vi "Continuous Swept-Sine MeasurementsV2.vi"() -> ()   [LabVIEW 2018]
doc: "Overview:\nThis VI demonstrates simultaneous frequency response, level, and distortion measurements using a discrete swept-sine technique. This example implements analog input and analog output with 'Finite Samples' sample mode which minimizes sensitivity to bandwidth issues that can cause run-time errors when performing continuous measurements. This VI also demonstrates how finite acquisitions can be read in a single large block or in a series of smaller reads.\n\nRequirements:\nLabVIEW Full Development System\nSound and Vibration Toolkit\n\nInstructions:\n1. Connect the DUT to the DSA device.\n2. Select the AO excitation channel, AI stimulus channel, and AI response channel.\n3. Run the VI.\n\nDetails:\nThis VI performs a swept sine measurement to obtain the root-mean-square (RMS) levels of the acquired stimulus and response, the frequency response of the device under test (DUT), and the harmonic distortion on the response channel. You specify the source and measurement parameters, and the swept sine VIs handle all the DAQ-specific controls required to perform the measurement. You have direct control over the source, input, averaging, and display parameters. You also specify the engineering units to use for the swept sine measurements.\n\nYou can view the time records of the acquired stimulus and response signals. From these graphs, you can see that the transition to the next test frequency always occurs at a zero crossing to minimize non-linear disturbances to the DUT. The RMS levels, frequency response, and harmonic distortion are shown on different tabs."
uses:
  <vilib>/sound2/lvsound2.llb/Sampling Mode.ctl
  <vilib>/sound2/lvsound2.llb/Sound Data Format.ctl
  <vilib>/Utility/error.llb/DialogType.ctl
  <vilib>/addons/_NISVFA/_Shared subVIs/Controls/svc_Window.ctl
  <vilib>/addons/_NISVFA/_Generation/Signal Generation/SV Signal/SV Signal.lvclass/SV Signal.ctl
  <vilib>/addons/_NISVFA/_Shared subVIs/Common/svc_Get Waveform Subset (Index).vi
  <vilib>/addons/_NISVFA/_Generation/Signal Generation/SV Signal/Write Leading Synchronization Pulse Enable.vi
  <vilib>/addons/_NISVFA/_Generation/Signal Generation/SV Signal/Write Ramp-Up.vi
  <vilib>/addons/_NISVFA/_Generation/Signal Generation/SV Signal/Write Ramp-Down.vi
  <vilib>/addons/_NISVFA/_Shared subVIs/Common/svc_Get Array Subset (Index).vi
  <vilib>/addons/_NISVFA/_Shared subVIs/Common/svc_Coerce Index and Length.vi
  <vilib>/addons/_NISVFA/_Shared subVIs/Common/svc_Conditional Merge Error.vi
  <vilib>/addons/_NISVFA/_Generation/Signal Generation/SV Continuous Sweep/SV Continuous Sweep.lvclass
  C:/Program Files (x86)/National Instruments/LabVIEW 2018/vi.lib/addons/_NISVFA/_Generation/Signal Generation/SV Signal/SV Signal.lvclass
  <vilib>/addons/_NISVFA/_Generation/Signal Generation/SV Continuous Sweep/Configure Continuous Sweep.vi
  <vilib>/addons/_NISVFA/_Generation/Signal Generation/SV Signal/Write Ramp Parameters.vi
  <vilib>/addons/_NISVFA/_Generation/Signal Generation/SV Signal/Write DC Offset.vi
  <vilib>/addons/_NISVFA/_Generation/Signal Generation/SV Signal/Write Transition Profile.vi
  <vilib>/addons/_NISVFA/_Generation/Signal Generation/SV Signal/Write Pre-Measurement Settling Duration.vi
  <vilib>/addons/_NISVFA/_Generation/Signal Generation/SV Signal/Write Post-Measurement Settling Duration.vi
  <vilib>/sound2/lvsound2.llb/Sound Output Set Volume (Single).vi
  <vilib>/sound2/lvsound2.llb/Sound Output Write (DBL Single).vi
  <vilib>/sound2/lvsound2.llb/Sound Input Read (DBL).vi
  <vilib>/Waveform/WDTOps.llb/WDT Copy Waveform dt DBL.vi
  <vilib>/measure/maresamp.llb/Align N Waveforms (single shot).vi
  <vilib>/addons/_NISVFA/_Baseband FFT/SVFA FFT Spectrum (Complex) (1 Ch).vi
  <vilib>/addons/Sound and Vibration/svt_Single Tone Measurements/SVT Gain and Phase (Frequency).vi
  <vilib>/addons/Sound and Vibration/svt_Distortion/SVT THD and Harmonic Components (Frequency) (1 Ch).vi
  <vilib>/addons/_NISVFA/_Generation/Signal Generation/SV Signal/SV Signal.lvclass
  Program Files (x86)/National Instruments/LabVIEW 2018/examples/Sound and Vibration/SoundVib_Audio Examples.lvlib
  <vilib>/addons/Sound and Vibration/svt_Continuous Swept Sine/SoundVib_ContSweptSine.lvlib
  <vilib>/addons/Sound and Vibration/svt_Distortion/SoundVib_Distortion.lvlib
  <vilib>/addons/Sound and Vibration/svt_Single Tone Measurements/SoundVib_SingleTone.lvlib
  <vilib>/measure/NI_MAPro.lvlib
panel:
  in  "device In":u32
  in  "device Out":u32=1
  out "Magnitude":cluster{"frequency":dbl[], "magnitude":dbl[]}(graph)
  out "Phase":cluster{"frequency":dbl[], "magnitude":dbl[]}(graph)
  out "THD":cluster{"frequency":dbl[], "THD":dbl[]}(graph)
  out "Waveform Graph":waveform(dbl)[](graph)
  out "error aP":errorcluster
  in  "Samples/Sec":dbl=44100.0
  out "test time":u32 format="%.0f ms"
  out "error Mic":errorcluster
  out "error Spkr":errorcluster
  in  "DC offset":dbl format="%.2f V"
  in  "amplitude":dbl=1.0 format="%.2p V"
  in  "frequency range":cluster{"start":dbl, "stop":dbl}={"start"=20000.0, "stop"=40.0} {"stop" min=0.0 format="%.2f Hz"; "start" min=0.0 format="%.2f Hz"}
  in  "duration":dbl=3.0 min=0.0 format="%.2f s"
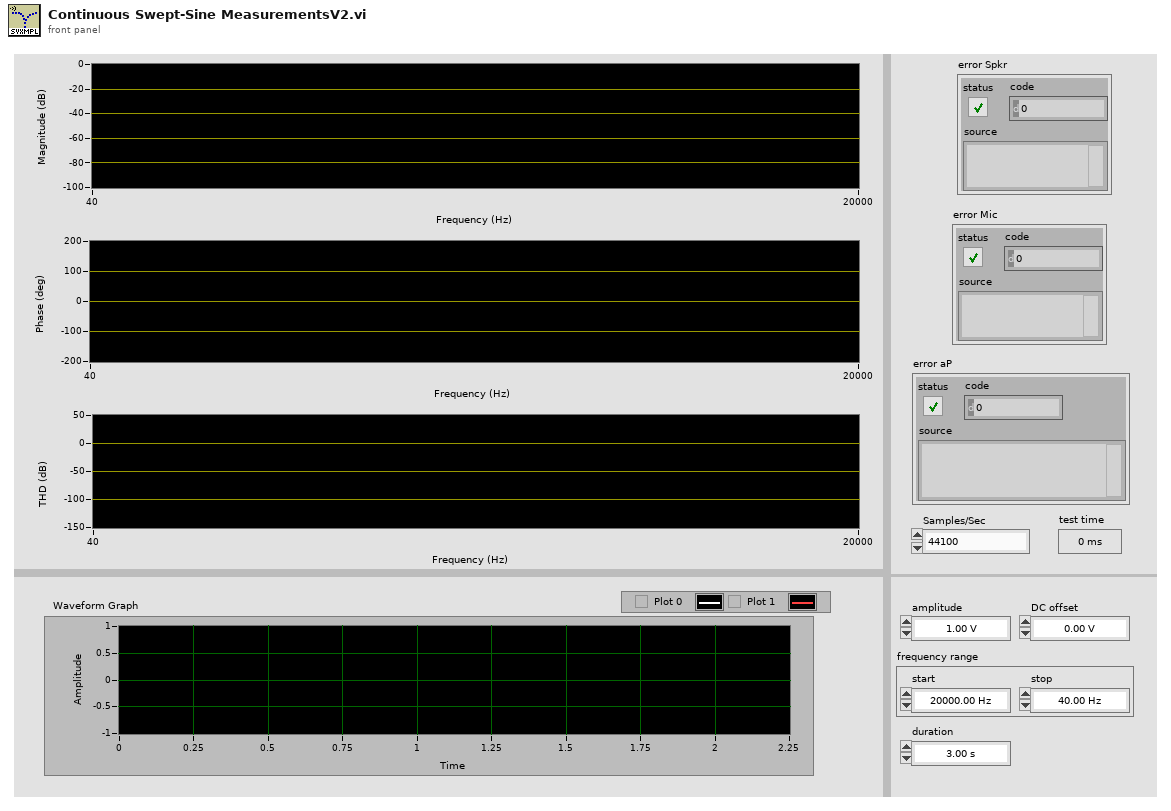
[diagram p1: front panel]
types:
  T1 = typedef "DialogType.ctl" = u16
  T2 = typedef "Sound Data Format.ctl" = cluster{"sample rate (S/s)":dbl, "number of channels":i32, "bits per sample":i32}
  T3 = typedef "Sampling Mode.ctl" = i32
  T4 = cluster{"start frequency":dbl, "stop frequency":dbl, "number of steps":i32}
  T5 = cluster{"profile":enum16{"Linear", "Half cosine"}, "durations [s]":cluster{"ramp-up":dbl, "transition":dbl, "ramp-down":dbl}}
  T6 = typedef "Sound Output Task ID.ctl" = u32
  T7 = typedef "Sound Input Task ID.ctl" = u32
  T8 = cluster{"averaging mode":enum16{"No averaging", "Vector averaging", "RMS averaging", "Peak hold"}, "weighting mode":enum16{"Linear", "Exponential"}, "number of averages":u32, "linear mode":enum16{"One shot", "Auto restart"}}
  T9 = typedef "svc_Window.ctl" = u32
  T10 = typedef "svc_Spectrum Info.ctl" = cluster{"channel name":string, "description":string, "x-axis units":T11, "spectral info":cluster{"spectrum type":T12, "linear/dB":enum16{"linear", "dB"}, "window":u16, "window size":i32, "FFT size":i32}, "engineering units":T13, "custom label":string, "dB reference [EU]":dbl, "peak units":enum16{"rms", "peak", "peak-peak"}, "weighting filter":T14, "spectral density?":bool, "unit label":string, "spectrum skewed?":bool, "complimentary spectrum units":T15}
  T11 = typedef "svc_X-Axis Units.ctl" = u16
  T12 = typedef "svc_Spectrum Type.ctl" = enum16{"FFT Spectrum [complex]", "Amplitude [Magnitude]", "Power [Magnitude^2]", "Cross Spectrum [complex]", "Frequency Response [Complex]"}
  T13 = typedef "svc_Engineering Units Text Ring.ctl" = u16
  T14 = typedef "svc_Weighting Filter Text Ring.ctl" = u16
  T15 = typedef "svc_Complimentary Spectrum Units.ctl" = enum16{"none", "radians", "degrees", "cycles", "imaginary"}
  T16 = cluster{"complex spectrum response":cluster{"f0":dbl, "df":dbl, "complex spectrum":cdb[]}, "spectrum info":T10}
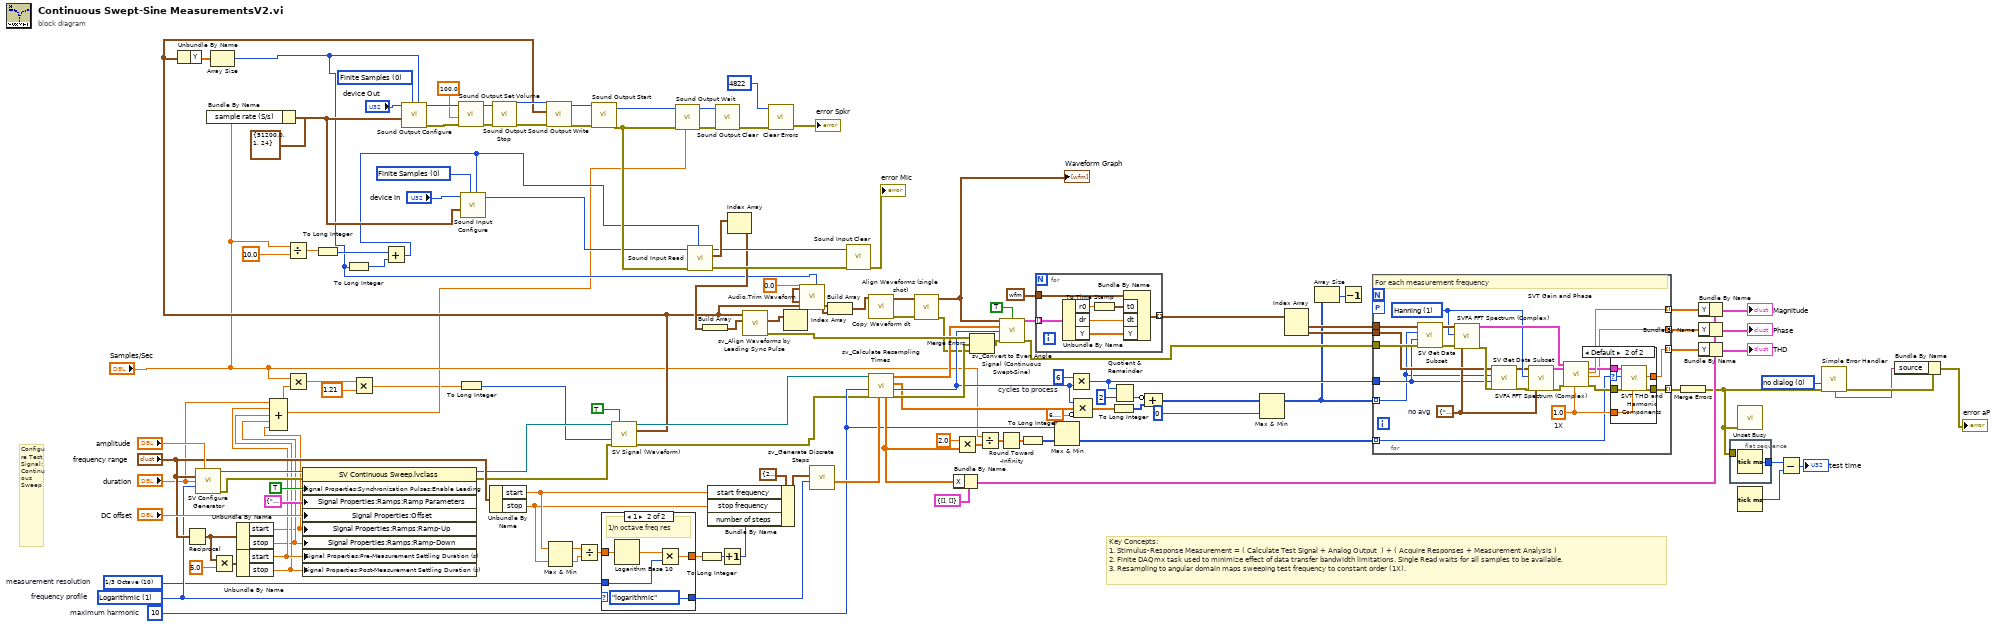
[diagram p0: block diagram]
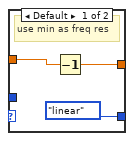
[diagram p2: hidden frame]
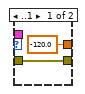
[diagram p3: hidden frame]
diagram:
  w22 = T1 0 items=["no dialog", "OK message", "continue or stop message", "OK message + warnings", "continue/stop + warnings"] ("type of dialog (OK msg:1)")
  w63 = T3 0 items=["Finite Samples", "Continuous Samples"] ("sample mode")
  w65 = T3 0 items=["Finite Samples", "Continuous Samples"] ("sample mode")
  w72 = u16 10 items=["1/3 Octave"=10, "1/6 Octave"=20, "1/12 Octave"=40, "1/24 Octave"=80, "1/48 Octave"=160]  # measurement resolution
  w86 = u16 1 items=["Linear", "Logarithmic"]  # frequency profile
  w108 = 6  # cycles to process
  w75 = 10  # maximum harmonic
  # "Key Concepts:\n1. Stimulus-Response Measurement = ( Calculate Test Signal + Analog Output  ) + ( Acquire Responses + Measurement Analysis )\n2. Finite DAQmx task used to minimize effect of data transfer bandwidth limitations. Single Read waits for all samples to be available.\n3. Resampling to angular domain maps sweeping test frequency to constant order (1X)."
  # "Configure Test Signal: \nContinuous Sweep"
  n1 = Reciprocal(x="frequency range") -> (1/x=w99:cluster{"start":dbl, "stop":dbl})
  n2 = call-poly <vilib>:"SV Configure Generator.vi"("amplitude"="amplitude", "frequency range [Hz]"="frequency range", "duration [s]"="duration", "profile"=w86) -> ("signal configuration"=w135:refnum<class "SV Continuous Sweep.lvclass">, "error out"=w132:errorcluster)  [unwired: 10 in]
  n3 = Bundle By Name(cluster=T2 {"sample rate (S/s)"=51200.0, "number of channels"=1, "bits per sample"=24} ("sound format"), "sample rate (S/s)"="Samples/Sec") -> (w57:T2)
  n4 = Multiply(x=w99, y=5.0 ("stop")) -> (x*y=w100:cluster{"start":dbl, "stop":dbl})
  n5 = Unbundle By Name(w99) -> ("start"=w5:dbl, "stop"=w6:dbl)
  n6 = Unbundle By Name(w100) -> ("start"=w9:dbl, "stop"=w8:dbl)
  n7 = Compound Arithmetic op=ADD("duration", w9, w8, w6, w5) -> (w10:dbl)
  n8 = Divide(x="Samples/Sec", y=10.0) -> (x/y=w54:dbl)
  n9 = Multiply(x="Samples/Sec", y=w10) -> (x*y=w4:dbl)
  n10 = property class="SV Continuous Sweep.lvclass"(reference=w135, error in=w132, "Signal Properties:Synchronization Pulses:Enable Leading"=TRUE ("Synchronization Pulses:Enable Leading"), "Signal Properties:Ramps:Ramp Parameters"=T5 {"profile"=enum."Half cosine", "durations [s]"={"ramp-up"=0.01, "transition"=0.0, "ramp-down"=0.01}} ("Ramp Parameters"), "Signal Properties:Offset"="DC offset", "Signal Properties:Ramps:Ramp-Up"=w5, "Signal Properties:Ramps:Ramp-Down"=w6, "Signal Properties:Pre-Measurement Settling Duration (s)"=w9, "Signal Properties:Post-Measurement Settling Duration (s)"=w8) -> (reference out=w35:refnum<class "SV Continuous Sweep.lvclass">, error out=w1:errorcluster)
  n11 = To Long Integer(number=w54) -> (32bit integer=w53:i32)
  n12 = Multiply(x=w4, y=1.21) -> (x*y=w2:dbl)
  n13 = To Long Integer(number=w2) -> (32bit integer=w7:i32)
  n14 = Unbundle By Name("frequency range") -> ("start"=w90:dbl, "stop"=w89:dbl)
  n15 = Max & Min(x=w90, y=w89) -> (max(x,y)=w95:dbl, min(x,y)=w94:dbl)
  n16 = Divide(x=w95, y=w94) -> (x/y=w93:dbl)
  n17 = case shown="1" w86 {
    tunnel: w93 -> [w137 w143]
    tunnel: [w136 w141] -> w92
    tunnel: [enum16{"linear", "logarithmic"}."linear" ("spacing") enum16{"linear", "logarithmic"}."logarithmic" ("spacing")] -> w87
    tunnel: w72 -> [_ w139]
    frame Default {
      # "use min as freq res"
      n18 = Decrement(x=w137) -> (x-1=w136:dbl)
    }
    frame 1 {
      # "1/n octave freq res"
      n19 = Logarithm Base 10(1:w143) -> (0:w142:dbl)
      n20 = Multiply(x=w142, y=w139) -> (x*y=w141:dbl)
    }
  }
  n21 = call-dynamic "SV Signal (Waveform).vi"("signal configuration"=w35, "reset"=TRUE, "samples"=w7, "error in (no error)"=w1) -> ("signal configuration"=w33:refnum<class "SV Continuous Sweep.lvclass">, "output waveform"=w31:waveform(dbl), "error out"=w32:errorcluster)  [unwired: 6 in, 3 out]
  n22 = Unbundle By Name(w31) -> ("Y"=w56:dbl[])
  n23 = Array Size(array=w56) -> (size(s)=w26:i32)
  n24 = To Long Integer(number=w26) -> (32bit integer=w52:i32)
  n25 = Add(x=w53, y=w52) -> (x+y=w42:i32)
  n26 = call <vilib>:"Sound Output Configure.vi"("number of samples/ch"=w26, "sample mode"=w65, "sound format"=w57, "device ID"="device Out") -> ("error out"=w69:errorcluster, "task ID"=w68:T6)  [unwired: 6 in]
  n27 = call-poly <vilib>:"Sound Output Set Volume.vi"("error in (no error)"=w69, "volume"=100.0, "task ID"=w68) -> ("error out"=w61:errorcluster, "task ID out"=w62:T6)  [unwired: 7 in]
  n28 = call <vilib>:"Sound Input Configure.vi"("number of samples/ch"=w42, "sample mode"=w63, "sound format"=w57, "device ID"="device In") -> ("task ID"=w41:T7)  [unwired: 6 in, 1 out]
  n29 = call <vilib>:"Sound Output Stop.vi"("error in (no error)"=w61, "task ID"=w62) -> ("error out"=w59:errorcluster, "task ID out"=w60:T6)  [unwired: 8 in]
  n30 = call-poly <vilib>:"Sound Output Write.vi"("error in (no error)"=w59, "data"=w31, "task ID"=w60) -> ("error out"=w43:errorcluster, "task ID out"=w44:T6)  [unwired: 7 in]
  n31 = call <vilib>:"Sound Output Start.vi"("error in (no error)"=w43, "task ID"=w44) -> ("error out"=w48:errorcluster, "task ID out"=w49:T6)  [unwired: 8 in]
  n32 = call <vilib>:"Sound Output Wait.vi"("timeout (sec)"=w10, "error in (no error)"=w48, "task ID"=w49) -> ("error out"=w51:errorcluster, "task ID out"=w50:T6)  [unwired: 7 in]
  n33 = call-poly <vilib>:"Sound Input Read.vi"("number of samples/ch"=w42, "error in (no error)"=w48, "task ID"=w41) -> ("error out"=w39:errorcluster, "data"=w47:waveform(dbl)[], "task ID out"=w40:T7)  [unwired: 6 in]
  n34 = To Long Integer(number=w92) -> (32bit integer=w91:i32)
  n35 = call <vilib>:"Sound Output Clear.vi"("error in (no error)"=w51, "task ID"=w50) -> ("error out"=w46:errorcluster)  [unwired: 9 in]
  n36 = Increment(x=w91) -> (x+1=w88:i32)
  n37 = Bundle By Name(cluster=T4 {"start frequency"=20.0, "stop frequency"=20000.0, "number of steps"=100} ("sweep frequencies"), "start frequency"=w90, "stop frequency"=w89, "number of steps"=w88) -> (w96:T4)
  n38 = Index Array(array=w47) -> (element=w38:waveform(dbl))  [unwired: 1 in]
  n39 = Build Array(w38) -> (w70:waveform(dbl)[])
  n40 = call "sv_Align Waveforms by Leading Sync Pulse.vi"("response signals"=w70, "alignment reference signal"=w31) -> ("error out"=w118:errorcluster, "aligned signals"=w30:waveform(dbl)[])  [unwired: 5 in, 3 out]
  n41 = call <vilib>:"Clear Errors.vi"("error in (no error)"=w46, "specific error code to clear (0: all)"=4822) -> ("error out"=→"error Spkr":errorcluster)  [unwired: 4 in, 1 out]
  n42 = Index Array(array=w30) -> (element=w29:waveform(dbl))  [unwired: 1 in]
  n43 = call "Audio.Trim Waveform.vi"("Len"=w26, "Max Delay"=0.0, "Data In"=w29) -> ("Data Out"=w27:waveform(dbl))  [unwired: 8 in]
  n44 = call <vilib>:"sv_Generate Discrete Steps.vi"("spacing"=w87, "steps"=w96) -> ("frequency list"=w83:dbl[])  [unwired: 8 in, 1 out]
  n45 = Build Array(w31, w27) -> (w16:waveform(dbl)[])
  n46 = call <vilib>:"Sound Input Clear.vi"("error in (no error)"=w39, "task ID"=w40) -> ("error out"=→"error Mic":errorcluster)  [unwired: 9 in]
  n47 = call-poly <vilib>:"Copy Waveform dt.vi"("waveforms in"=w16) -> ("error out"=w17:errorcluster, "waveforms out"=w18:waveform(dbl)[])  [unwired: 9 in]
  n48 = call "sv_Calculate Resampling Times.vi"("measurement frequencies in (Hz)"=w83, "error in"=w32, "maximum harmonic"=w75, "continuous sweep configuration"=w33) -> ("error out"=w117:errorcluster, "samples/rev"=w107:i32, "measurement phases (rad)"=w84:dbl[], "resampling times (s)"=w85:dbl[], "measurement frequencies (Hz)"=w76:dbl[])  [unwired: 1 in, 2 out]
  n49 = call-poly <vilib>:"Align Waveforms (single shot).vi"("error in (no error)"=w17, "waveforms in"=w18) -> ("error out"=w14:errorcluster, "aligned waveforms out"=w15:waveform(dbl)[])  [unwired: 8 in]
  "Waveform Graph" <- w15
  n50 = Bundle By Name(cluster=cluster{"X":dbl[], "Y":dbl[]} {"X"=[], "Y"=[]} ("THD vs Amplitude"), "X"=w76) -> (w125:cluster{"X":dbl[], "Y":dbl[]})
  n51 = Multiply(x=2.0 ("y"), y=w76) -> (x*y=w80:dbl[])
  n52 = Merge Errors(w118, w117, w14) -> (w116:errorcluster)
  n53 = Divide(x="Samples/Sec", y=w80) -> (x/y=w79:dbl[])
  n54 = Round Toward -Infinity(1:w79) -> (0:w78:dbl[])
  n55 = call <vilib>:"sv_Convert to Even Angle Signal (Continuous Swept-Sine).vi"("scaled signals [EU]"=w15, "reset? (F)"=TRUE, "new sample time [s]"=w85, "new samples/rev"=w107, "error in (no error)"=w116) -> ("even-angle signals"=w121:cluster{"r0":dbl, "dr":dbl, "Y":dbl[]}[], "error out"=w71:errorcluster)  [unwired: 6 in, 3 out]
  n56 = To Long Integer(number=w78) -> (32bit integer=w74:i32[])
  n57 = for {
    tunnel: w121 -> [w150] mode=indexing
    tunnel: waveform(dbl) {"t0"=timestamp(0 s since 1904-01-01), "dt"=1.0, "Y"=[]} ("waveform out") -> [w145]
    tunnel: [w144] -> w13 mode=indexing
    n58 = Unbundle By Name(w150) -> ("r0"=w149:dbl, "dr"=w147:dbl, "Y"=w146:dbl[])
    n59 = To Time Stamp(1:w149) -> (0:w148:timestamp)
    n60 = Bundle By Name(cluster=w145, "t0"=w148, "dt"=w147, "Y"=w146) -> (w144:waveform(dbl))
  }
  n61 = Max & Min(x=w75, y=w74) -> (min(x,y)=w73:i32[])  [unwired: 1 out]
  n62 = Multiply(x=w108, y=w107) -> (x*y=w105:i32)
  n63 = Compound Arithmetic op=MULTIPLY(w107, w84, invert 6.283185307179586) -> (w82:dbl[])
  n64 = To Long Integer(number=w82) -> (32bit integer=w104:i32[])
  n65 = Quotient & Remainder(x=w105, y=2 ("x")) -> (floor(x/y)=w106:i32)  [unwired: 1 out]
  n66 = Compound Arithmetic op=ADD(invert w106, w104) -> (w102:i32[])
  n67 = Max & Min(x=w102, y=0 ("x")) -> (max(x,y)=w25:i32[])  [unwired: 1 out]
  n68 = Index Array(array=w13) -> (element #1=w114:waveform(dbl), element #2=w113:waveform(dbl))  [unwired: 2 in]
  n69 = Array Size(array=w25) -> (size(s)=w24:i32)
  n70 = Decrement(x=w24) -> ()  [unwired: 1 out]
  n71 = for {
    tunnel: w71 -> [w173]
    tunnel: [w167] -> w115 mode=indexing
    tunnel: [w166] -> w112 mode=indexing
    tunnel: w114 -> [w165]
    tunnel: w113 -> [w164]
    tunnel: [w156] -> w110 mode=indexing
    tunnel: [w155] -> w111 mode=indexing
    tunnel: w105 -> [w154]
    tunnel: w25 -> [w153] mode=indexing
    tunnel: w73 -> [w151] mode=indexing
    workers-P: _ -> [_]
    w152 = 1.0  # 1X
    w157 = T8 {"averaging mode"=enum."No averaging", "weighting mode"=enum."Exponential", "number of averages"=10, "linear mode"=enum."One shot"}  # no avg
    w168 = T9 1 items=["None"=0, "Hanning"=1, "Hamming"=2, "Blackman-Harris"=3, "Exact Blackman"=4, "Blackman"=5, "Flat Top"=6, "4 Term B-Harris "=7, "7 Term B-Harris"=8, "Low Sidelobe"=9, "Force"=64, "Exponential"=65, "Blackman Nuttall"=11, "Triangle"=30, "Bartlett-Hanning"=31, "Bohman"=32, "Parzen"=33, "Welch"=34, "Kaiser"=60, "Dolph-Chebyshev"=61, "Gaussian"=62] ("window")
    # "For each measurement frequency"
    n72 = call-poly <vilib>:"SV Get Data Subset.vi"("error in (no error)"=w173, "length (-1 = all)"=w154, "start index (0)"=w153, "waveform in"=w165) -> ("error out"=w171:errorcluster, "waveform subset"=w172:waveform(dbl))  [unwired: 2 in, 4 out]
    n73 = call-poly <vilib>:"SVFA FFT Spectrum (Complex).vi"("scaled signal [EU]"=w172, "window"=w168, "error in"=w171, "averaging parameters"=w157) -> ("complex spectrum"=w169:T16, "error out"=w170:errorcluster)  [unwired: 12 in, 2 out]
    n74 = call-poly <vilib>:"SV Get Data Subset.vi"("error in (no error)"=w170, "length (-1 = all)"=w154, "start index (0)"=w153, "waveform in"=w164) -> ("error out"=w162:errorcluster, "waveform subset"=w163:waveform(dbl))  [unwired: 2 in, 4 out]
    n75 = call-poly <vilib>:"SVFA FFT Spectrum (Complex).vi"("scaled signal [EU]"=w163, "window"=w168, "error in"=w162, "averaging parameters"=w157) -> ("complex spectrum"=w159:T16, "error out"=w158:errorcluster)  [unwired: 12 in, 2 out]
    n76 = call-poly <vilib>:"SVT Gain and Phase.vi"("complex spectrum\nstimulus X"=w169, "complex spectrum\nresponse Y"=w159, "error in (no error)"=w158, "expected fundamental frequency [Hz]"=w152) -> ("dup complex spectrum\nresponse Y"=w161:T16, "gain"=w166:dbl, "phase lag"=w155:dbl, "error out"=w160:errorcluster)  [unwired: 8 in, 4 out]
    n77 = case shown="Default" w151 {
      selector: w151 -> [_ w176]
      tunnel: [w175 w181] -> w167
      tunnel: w161 -> [_ w180]
      tunnel: w160 -> [w175 w179]
      tunnel: [-120.0 ("THD") w178] -> w156
      tunnel: w152 -> [_ w177]
      frame ..1 {
      }
      frame Default {
        n78 = call-poly <vilib>:"SVT THD and Harmonic Components.vi"("complex spectrum"=w180, "maximum harmonic"=w176, "error in (no error)"=w179, "expected fundamental frequency [Hz]"=w177) -> ("THD"=w178:dbl, "error out"=w181:errorcluster)  [unwired: 8 in, 6 out]
      }
    }
  }
  n79 = Merge Errors(w115) -> (w23:errorcluster)
  n80 = Bundle By Name(cluster=w125, "Y"=w112) -> (→"Magnitude":cluster{"X":dbl[], "Y":dbl[]})
  n81 = Bundle By Name(cluster=w125, "Y"=w111) -> (→"Phase":cluster{"X":dbl[], "Y":dbl[]})
  n82 = Bundle By Name(cluster=w125, "Y"=w110) -> (→"THD":cluster{"X":dbl[], "Y":dbl[]})
  n83 = flat-sequence {
    tunnel: [w182] -> w124
    tunnel: w23 -> [_]
    frame #0 {
      n84 = Tick Count (ms)() -> (millisecond timer value=w182:u32)
    }
  }
  n85 = call <vilib>:"Unset Busy.vi"("error in (no error)"=w23) -> ()  [unwired: 10 in, 1 out]
  n86 = Tick Count (ms)() -> (millisecond timer value=w122:u32)
  n87 = Subtract(x=w124, y=w122) -> (x-y=→"test time":u32)
  n88 = call <vilib>:"Simple Error Handler.vi"("type of dialog (OK msg:1)"=w22, "error in (no error)"=w23) -> ("error out"=w21:errorcluster, "message"=w20:string)  [unwired: 3 in, 3 out]
  n89 = Bundle By Name(cluster=w21, "source"=w20) -> (→"error aP":errorcluster)
